vi "_script_fix_Find Event Stucture Ref vi.vi"   [LabVIEW 2014]
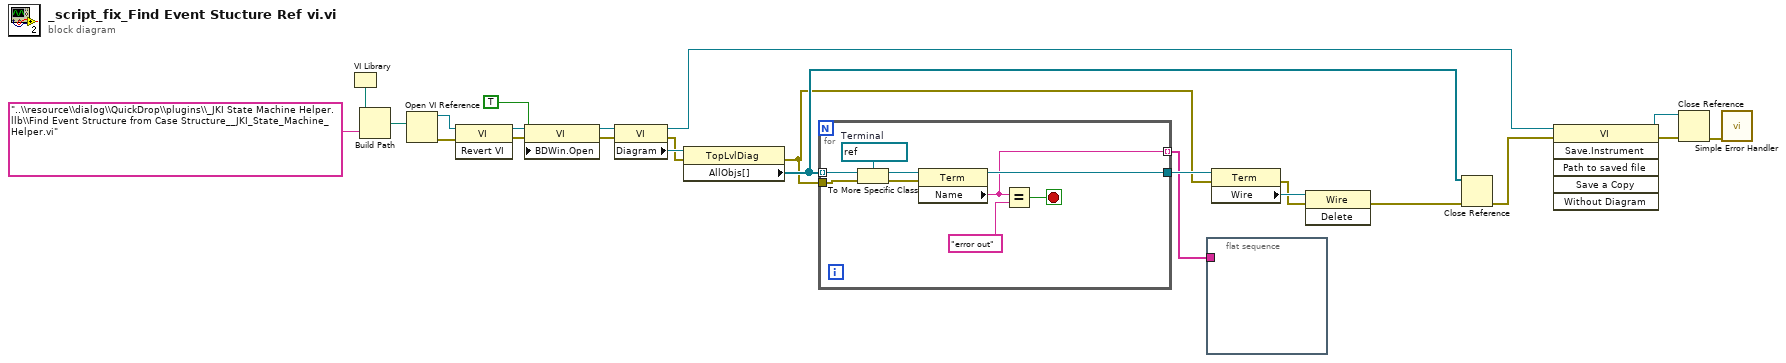
[diagram p0: block diagram]
diagram:
  n1 = VI Library() -> (path=w22:path)
  n2 = Build Path(base path=w22, name or relative path="..\\resource\\dialog\\QuickDrop\\plugins\\_JKI State Machine Helper.llb\\Find Event Structure from Case Structure__JKI_State_Machine_Helper.vi") -> (appended path=w20:path)
  n3 = Open VI Reference(vi path=w20) -> (vi reference=w23:refnum<vi>, error out=w24:errorcluster)  [unwired: 5 in]
  n4 = invoke class="VI" method="Revert VI"(reference=w23, error in=w24) -> (reference out=w16:refnum<vi>, error out=w15:errorcluster)  [unwired: 1 in, 1 out]
  n5 = property class="VI"(reference=w16, error in=w15, "BDWin.Open"=TRUE ("Block Diagram Window:Open")) -> (reference out=w14:refnum<vi>, error out=w13:errorcluster)
  n6 = property class="VI"(reference=w14, error in=w13) -> (reference out=w6:refnum<vi>, error out=w10:errorcluster, "Diagram"=w11:refnum<vi>)
  n7 = property class="TopLvlDiag"(reference=w11, error in=w10) -> (error out=w2:errorcluster, "AllObjs[]"=w4:refnum<vi>[])  [unwired: 1 out]
  n8 = for {
    tunnel: w4 -> [w33] mode=indexing
    tunnel: [w28] -> w9
    tunnel: w2 -> [w27]
    tunnel: [w25] -> w1 mode=indexing
    stop <- w29 stop-if-true
    w31 = refnum<vi> refnum  # Terminal
    n9 = To More Specific Class(target class=w31, reference=w33, error in=w27) -> (specific class reference=w32:refnum<vi>, error out=w26:errorcluster)
    n10 = property class="Term"(reference=w32, error in=w26) -> (reference out=w28:refnum<vi>, "Name"=w25:string)  [unwired: 1 out]
    n11 = Equal?(x=w25, y="error out") -> (x = y?=w29:bool)
  }
  n12 = flat-sequence {
    tunnel: w1 -> [_]
    frame #0 {
    }
  }
  n13 = property class="Term"(reference=w9, error in=w2) -> (error out=w7:errorcluster, "Wire"=w8:refnum<vi>)  [unwired: 1 out]
  n14 = invoke class="Wire" method="Delete"(reference=w8, error in=w7) -> (error out=w3:errorcluster)  [unwired: 1 in, 2 out]
  n15 = Close Reference(reference=w4, error in (no error)=w3) -> (error out=w5:errorcluster)
  n16 = invoke class="VI" method="Save.Instrument"(reference=w6, error in=w5) -> (reference out=w18:refnum<vi>, error out=w19:errorcluster)  [unwired: 4 in, 4 out]
  n17 = Close Reference(reference=w18, error in (no error)=w19) -> (error out=w17:errorcluster)
  n18 = call <vilib>:"Simple Error Handler.vi"("error in (no error)"=w17) -> ()  [unwired: 4 in, 5 out]
